vi "存储原始Data至TDMS.vi"(8 "error in (no error)":errorcluster caption="错误输入（无错误）", 11 "TDMS":refnum<k34>) -> (0 "error out":errorcluster caption="错误输出", 3 "TDMS 2":refnum<k34>)   [LabVIEW 2018]
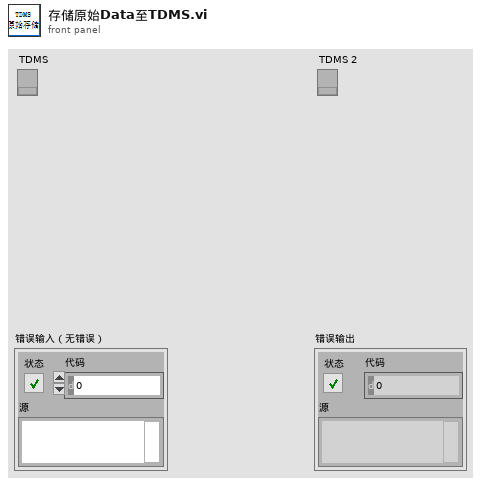
[diagram p1: front panel]
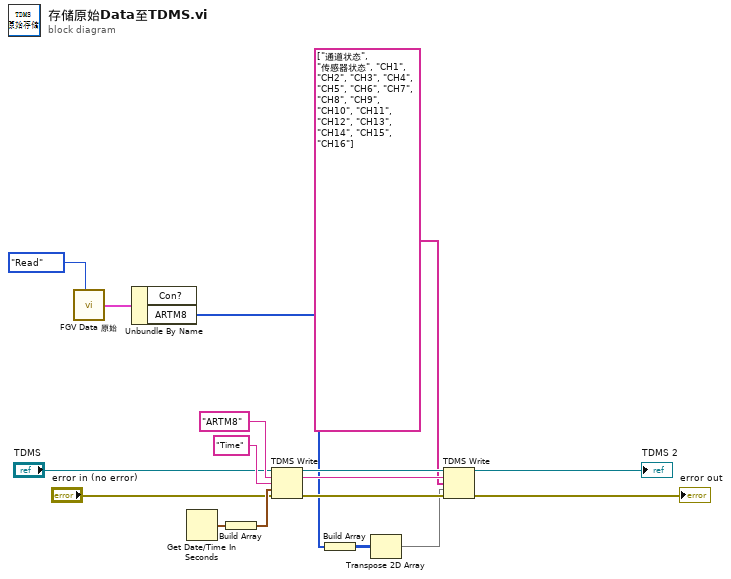
[diagram p0: block diagram]
diagram:
  n1 = call "FGV Data 原始.vi"("Action"=enum16{"Initial", "Read", "Write"}."Read") -> ("Data OUT"=w2:cluster{"Con?":bool, "ARTM8":u16[]})  [unwired: 9 in, 1 out]
  n2 = Unbundle By Name(w2) -> ("ARTM8"=w1:u16[])  [unwired: 1 out]
  n3 = Get Date/Time In Seconds() -> (seconds since 1Jan1904=w15:timestamp)
  n4 = Build Array(w15) -> (w14:timestamp[])
  n5 = TDMS Write(0:"TDMS", 5:"ARTM8" ("组名称输入（无标题）"), 7:"Time" ("组名称输入（无标题）"), 9:w14, 11:"error in (no error)") -> (4:w13:refnum<k34>, 6:w12:string, 15:w11:errorcluster)  [unwired: 1 in, 1 out]
  n6 = Build Array(w1) -> (w5:u16[][])
  n7 = Transpose 2D Array(2D array=w5) -> (transposed array=w4:u16[][])
  n8 = TDMS Write(0:w13, 5:w12, 7:string[] ["通道状态", "传感器状态", "CH1", "CH2", "CH3", "CH4", "CH5", "CH6", "CH7", "CH8", "CH9", "CH10", "CH11", "CH12", "CH13", "CH14", "CH15", "CH16"], 9:w4, 11:w11) -> (4:→"TDMS 2":refnum<k34>, 15:→"error out":errorcluster)  [unwired: 1 in, 2 out]
